vi "RunTest.vi"(8 "error in (no error)":errorcluster, 11 "reference in":refnum<class "Test_Base.lvclass">) -> (0 "error out":errorcluster, 1 "State":T1, 3 "reference in":refnum<class "Test_Base.lvclass">)   [LabVIEW 2022 SP3, in "Test_Base.lvlib" / "Test_Base.lvclass"]
uses:
  Test_Base.lvclass
  TestsState.ctl
  Components/TestView_Base.lvlibp/ViewStatus.ctl
  Components/MES_Base.lvlibp/MES_Base.lvclass
  Components/TestView_Base.lvlibp/TestView_Base.lvclass
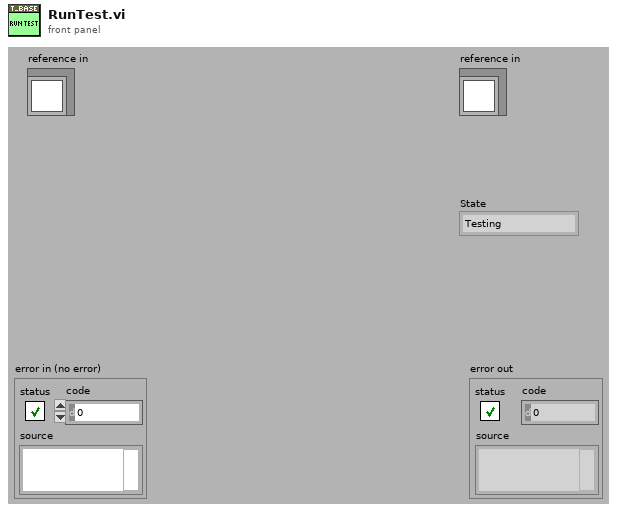
[diagram p1: front panel]
types:
  T1 = typedef "Test_Base.lvlib/Test_Base.lvclass/TestsState.ctl" = enum16{"Testing", "Pass", "Fail", "Abort", "Fault"}
  T2 = typedef "TestView_Base.lvlibp/TestView_Base.lvclass/ViewStatus.ctl" = enum16{"Testing", "Ready", "Logout", "Login", "PASS", "FAIL", "FAULT", "ABORTED"}
  T3 = typedef "Test_Base.lvlib/Test_Base.lvclass/ObjectAttributes.ctl" = cluster{"Config":T4, "UUTIndex":i32, "Serial":string, "Batch":string, "MES":refnum<class "MES_Base.lvclass">, "TestView":refnum<class "TestView_Base.lvclass">, "LoggedIn":bool, "Abort":bool}
  T4 = typedef "Test_Base.lvlib/Test_Base.lvclass/Config.ctl" = cluster{"ContinueOnFail":bool}
  T5 = cluster{"Code":string, "Name":string, "Description":string, "Group":string, "IsGroup":bool, "Tag":string, "Method":string, "Parrameter":string, "DataType":enum16{"NA", "String", "Boolean", "Int", "Dbl"}, "Value":variant, "Status":enum16{"Pending", "Pass", "Fail"}, "LimitLo":variant, "LimitHi":variant, "StringMatch":string, "BooleanMatch":bool, "DisplayFormat":string, "Units":string, "TestTime":dbl}
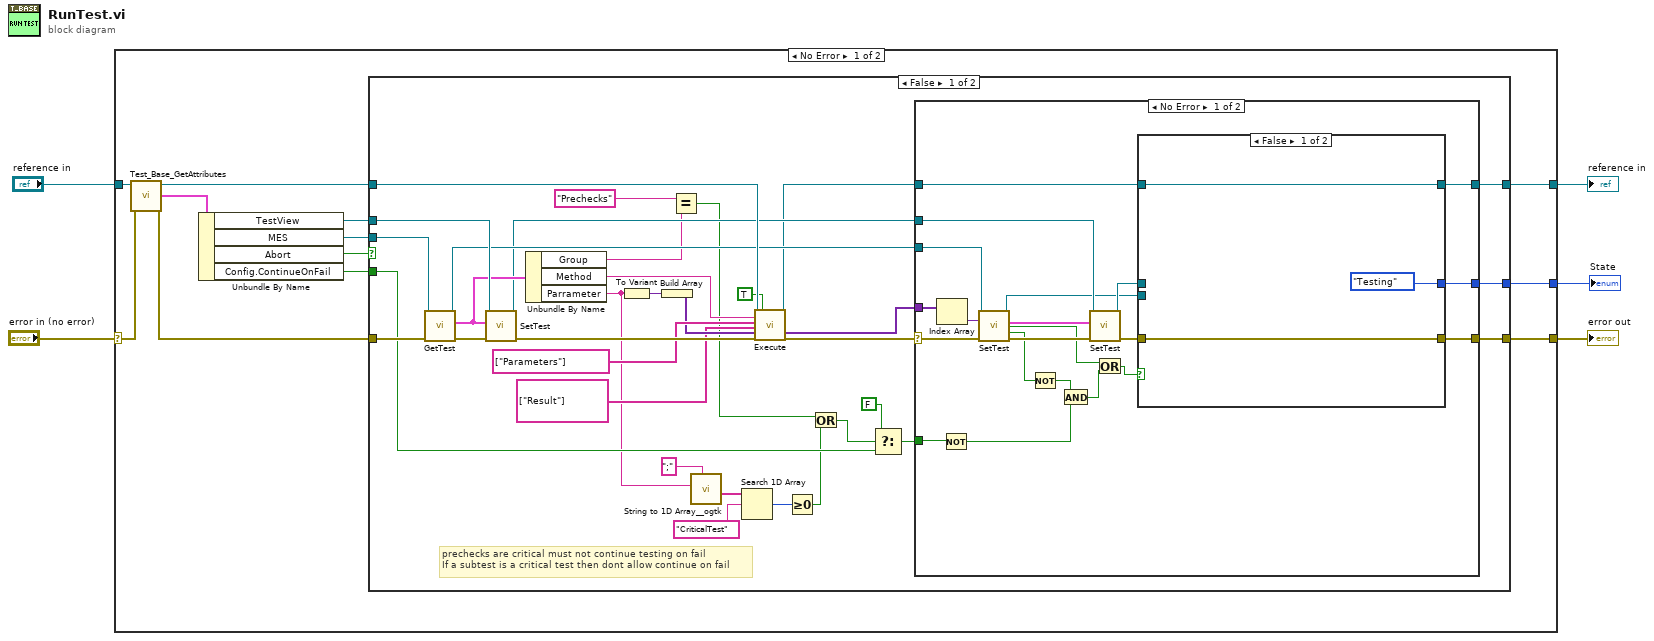
[diagram p0: block diagram]
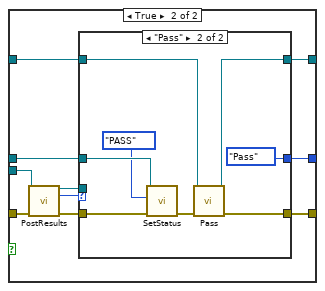
[diagram p2: hidden frame]
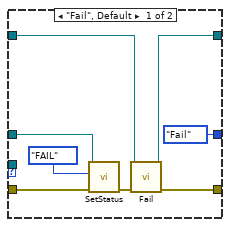
[diagram p3: hidden frame]
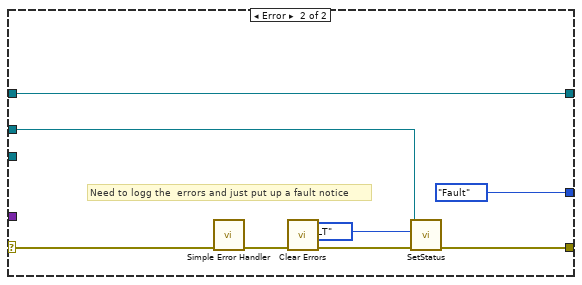
[diagram p4: hidden frame]
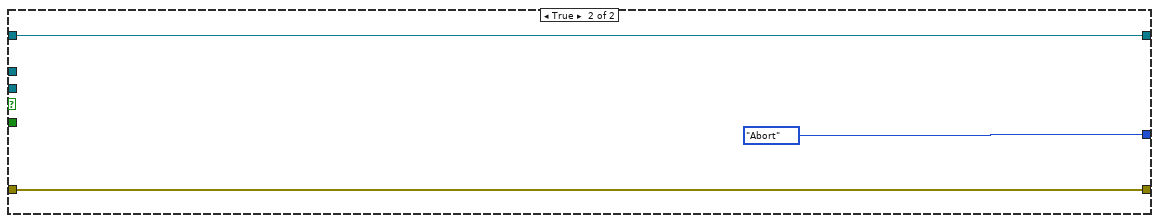
[diagram p5: hidden frame]
diagram:
  n1 = case shown="No Error" "error in (no error)" {
    selector: "error in (no error)" -> [w17 w114]
    tunnel: [w9 w114] -> w4
    tunnel: [w10 w113] -> w2
    tunnel: "reference in" -> [w15 w113]
    tunnel: [w7 _] -> w1
    frame No Error {
      n2 = call "Test_Base_GetAttributes.vi"("error in (no error)"=w17, "reference in"=w15) -> ("error out"=w14:errorcluster, "Data"=w16:T3, "reference out"=w11:refnum<class "Test_Base.lvclass">)  [unwired: 6 in, 1 out]
      n3 = Unbundle By Name(w16) -> ("TestView"=w12:refnum<class "TestView_Base.lvclass">, "MES"=w13:refnum<class "MES_Base.lvclass">, "Abort"=w8:bool, "Config.ContinueOnFail"=w6:bool)
      n4 = case shown="False" w8 {
        tunnel: w14 -> [w51 w111]
        tunnel: w13 -> [w49 _]
        tunnel: w12 -> [w48 _]
        tunnel: w11 -> [w46 w112]
        tunnel: [w34 w112] -> w10
        tunnel: [w33 w111] -> w9
        tunnel: [w31 TestsState."Abort" ("State")] -> w7
        tunnel: w6 -> [w27 _]
        frame False {
          # "prechecks are critical must not continue testing on fail\nIf a subtest is a critical test then dont allow continue on fail"
          n5 = call-dynamic "GetTest.vi"("error in (no error)"=w51, "reference in"=w49) -> ("error out"=w50:errorcluster, "Test"=w45:T5, "reference in"=w37:refnum<class "MES_Base.lvclass">)  [unwired: 7 in]
          n6 = call-dynamic "SetTest.vi"("error in (no error)"=w50, "Test"=w45, "reference in"=w48) -> ("error out"=w47:errorcluster, "reference in"=w36:refnum<class "TestView_Base.lvclass">)  [unwired: 7 in]
          n7 = Unbundle By Name(w45) -> ("Group"=w30:string, "Method"=w44:string, "Parrameter"=w24:string)
          n8 = To Variant(anything=w24) -> (Variant=w41:variant)
          n9 = Build Array(w41) -> (w40:variant[])
          n10 = Equal?(x="Prechecks", y=w30) -> (x = y?=w20:bool)
          n11 = call <userlib>:"String to 1D Array__ogtk.vi"("delimiter (Tab)"=";", "string"=w24) -> ("Array of Strings"=w23:string[])  [unwired: 9 in]
          n12 = Search 1D Array(1D array=w23, element="CriticalTest") -> (index of element=w21:i32)  [unwired: 1 in]
          n13 = call-dynamic "Execute.vi"("reference in"=w46, "cmd"=w44, "controls"=string[] ["Parameters"], "indicators"=string[] ["Result"] ("controls"), "control data"=w40, "error in (no error)"=w47, "must_exist"=TRUE) -> ("reference out"=w35:refnum<class "Test_Base.lvclass">, "indicator data"=w38:variant[], "error out"=w32:errorcluster)  [unwired: 8 in, 2 out]
          n14 = Greater Or Equal To 0?(x=w21) -> (x >= 0?=w18:bool)
          n15 = Or(x=w20, y=w18) -> (x .or. y?=w19:bool)
          n16 = Select(t=FALSE ("must_exist"), s=w19, f=w27) -> (s? t:f=w26:bool)
          n17 = case shown="No Error" w32 {
            selector: w32 -> [w60 w107]
            tunnel: w38 -> [w72 _]
            tunnel: w37 -> [w71 _]
            tunnel: w36 -> [w68 w102]
            tunnel: w35 -> [w63 w108]
            tunnel: [w62 w108] -> w34
            tunnel: [w61 w103] -> w33
            tunnel: [w59 TestsState."Fault" ("State")] -> w31
            tunnel: w26 -> [w58 _]
            frame No Error {
              n18 = Index Array(array=w72) -> (element=w70:variant)  [unwired: 1 in]
              n19 = Not(x=w58) -> (.not. x?=w54:bool)
              n20 = call-dynamic "SetTest.vi"("reference in"=w71, "Value"=w70, "error in (no error)"=w60) -> ("reference in"=w64:refnum<class "MES_Base.lvclass">, "Test"=w67:T5, "Complete"=w57:bool, "Pass"=w56:bool, "error out"=w69:errorcluster)  [unwired: 8 in]
              n21 = Not(x=w56) -> (.not. x?=w55:bool)
              n22 = And(x=w55, y=w54) -> (x .and. y?=w53:bool)
              n23 = call-dynamic "SetTest.vi"("error in (no error)"=w69, "Test"=w67, "reference in"=w68) -> ("error out"=w66:errorcluster, "reference in"=w65:refnum<class "TestView_Base.lvclass">)  [unwired: 7 in]
              n24 = Or(x=w57, y=w53) -> (x .or. y?=w52:bool)
              n25 = case shown="False" w52 {
                tunnel: w66 -> [w74 w85]
                tunnel: w65 -> [_ w76]
                tunnel: w64 -> [_ w84]
                tunnel: w63 -> [w75 w82]
                tunnel: [w75 w81] -> w62
                tunnel: [w74 w80] -> w61
                tunnel: [TestsState."Testing" ("State") w79] -> w59
                frame False {
                }
                frame True {
                  n26 = call-dynamic "PostResults.vi"("reference in"=w84, "error in (no error)"=w85) -> ("reference in"=w83:refnum<class "MES_Base.lvclass">, "Result"=w78:enum16{"Pending", "Pass", "Fail"}, "error out"=w77:errorcluster)  [unwired: 11 in]
                  n27 = case shown="\"Pass\"" w78 {
                    tunnel: w77 -> [w89 w97]
                    tunnel: w83 -> [_ _]
                    tunnel: w82 -> [w93 w101]
                    tunnel: [w92 w100] -> w81
                    tunnel: [w91 w99] -> w80
                    tunnel: [TestsState."Fail" ("State") TestsState."Pass" ("State")] -> w79
                    tunnel: w76 -> [w87 w95]
                    frame "Fail", Default {
                      n28 = call-dynamic "SetStatus.vi"("error in (no error)"=w89, "Status"=ViewStatus."FAIL", "reference in"=w87) -> ("error out"=w88:errorcluster)  [unwired: 7 in, 1 out]
                      n29 = call-dynamic "Fail.vi"("error in (no error)"=w88, "reference in"=w93) -> ("error out"=w91:errorcluster, "reference in"=w92:refnum<class "Test_Base.lvclass">)  [unwired: 8 in]
                    }
                    frame "Pass" {
                      n30 = call-dynamic "SetStatus.vi"("error in (no error)"=w97, "Status"=ViewStatus."PASS", "reference in"=w95) -> ("error out"=w96:errorcluster)  [unwired: 7 in, 1 out]
                      n31 = call-dynamic "Pass.vi"("error in (no error)"=w96, "reference in"=w101) -> ("error out"=w99:errorcluster, "reference in"=w100:refnum<class "Test_Base.lvclass">)  [unwired: 8 in]
                    }
                  }
                }
              }
            }
            frame Error {
              # "Need to logg the\t errors and just put up a fault notice"
              n32 = call <vilib>:"Simple Error Handler.vi"("error in (no error)"=w107) -> ("error out"=w106:errorcluster)  [unwired: 4 in, 4 out]
              n33 = call <vilib>:"Clear Errors.vi"("error in (no error)"=w106) -> ("error out"=w104:errorcluster)  [unwired: 5 in, 1 out]
              n34 = call-dynamic "SetStatus.vi"("error in (no error)"=w104, "Status"=ViewStatus."FAULT", "reference in"=w102) -> ("error out"=w103:errorcluster)  [unwired: 7 in, 1 out]
            }
          }
        }
        frame True {
        }
      }
    }
    frame Error {
    }
  }
  "error out" <- w4
  "reference in" <- w2
  "State" <- w1
